vi "read_nmt_state.vi"(11 "node":u8) -> (3 "return":u8)   [LabVIEW 2011]
uses:
  canopen_dll_master.dll
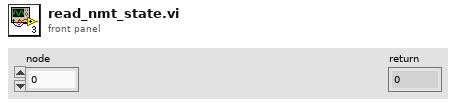
[diagram p1: front panel]
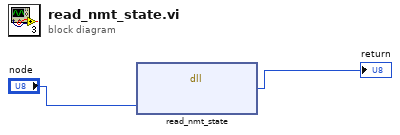
[diagram p0: block diagram]
diagram:
  n1 = dll-call lib="canopen_dll_master.dll" fn="read_nmt_state"("node"="node") -> ("return type"=→"return":u8)  [unwired: 4 in, 2 out]
